vi "Zufalls(Musik-)auswahl.vi"() -> ()   [LabVIEW 2010]
uses:
  <vilib>/gmath/statdist.llb/Random Permutation.vi
  <vilib>/gmath/NI_Gmath.lvlib
panel:
  in  "start":i32 caption="Start"
  out "ausgelassene":i32
  out "wiederholungen":i32
  in  "seed":i32 caption="Startwert"
  in  "reset":bool caption="Zurücksetzen"
  in  "Playlist 2":i32(listbox) caption="Playlist"
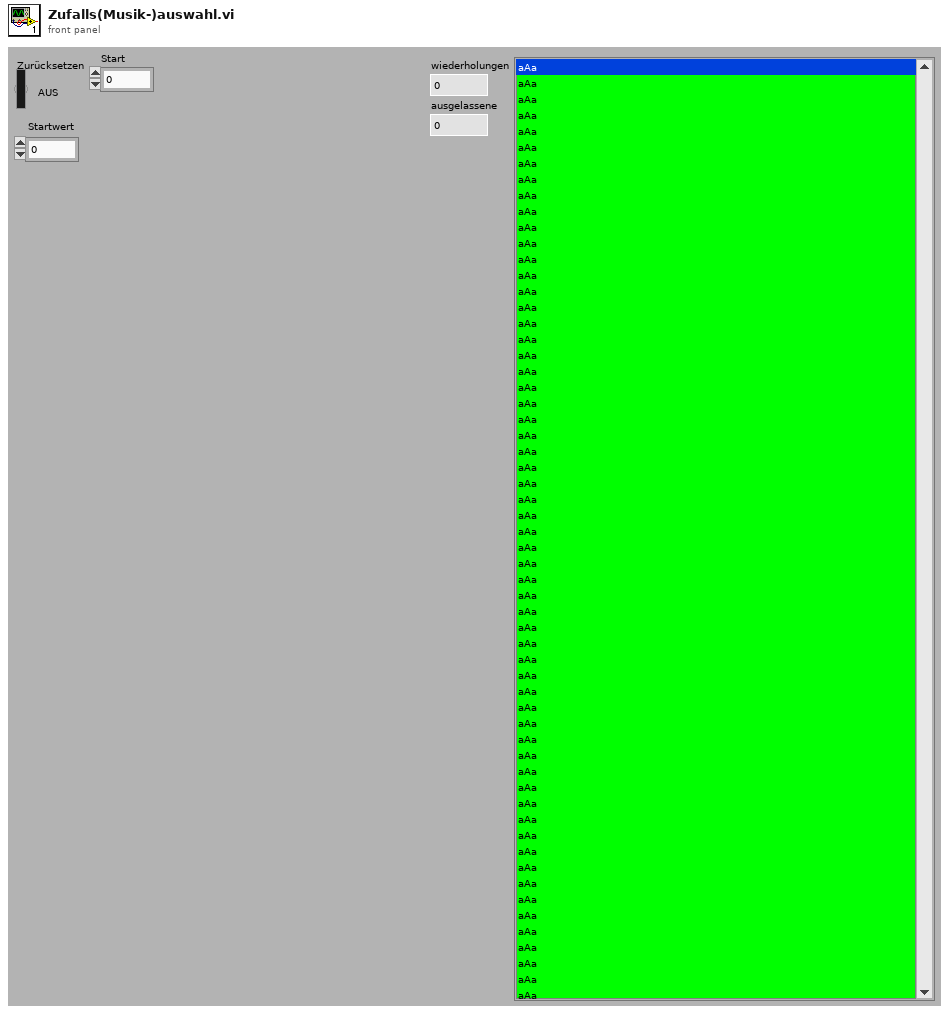
[diagram p1: front panel]
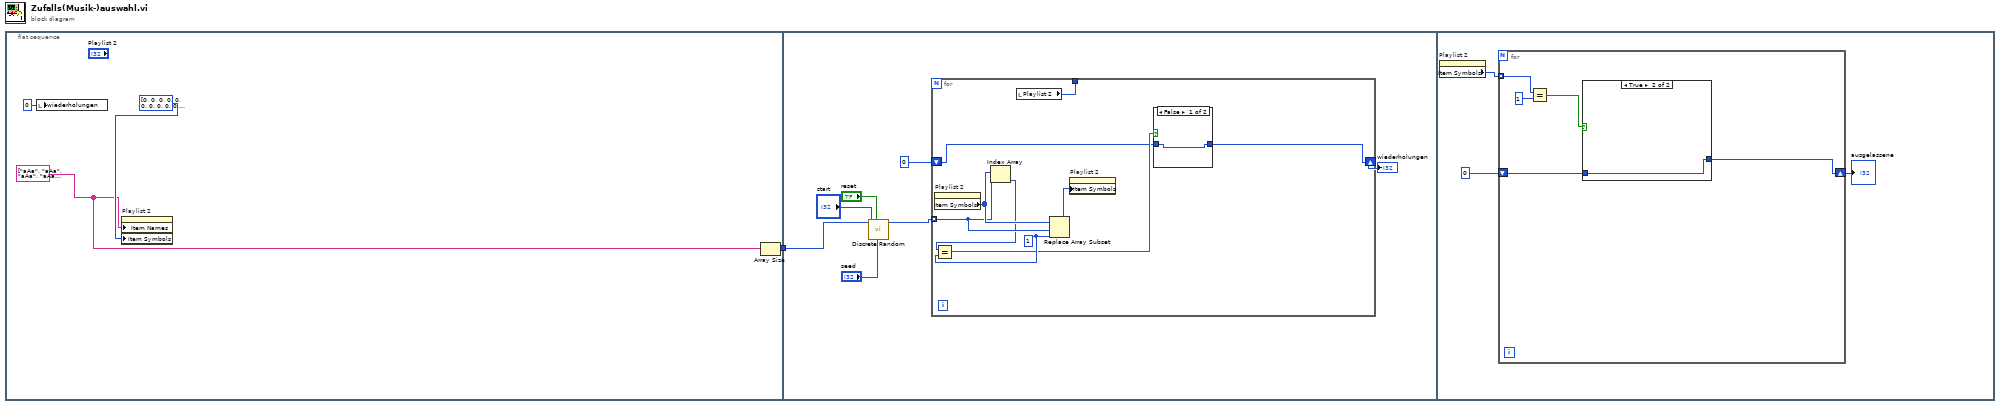
[diagram p0: block diagram]
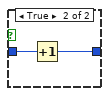
[diagram p2: hidden frame]
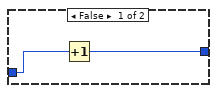
[diagram p3: hidden frame]
diagram:
  n1 = flat-sequence {
    tunnel: [w5] -> w1
    tunnel: w1 -> [w7]
    frame #0 {
      w2 = string[] ["aAa", "aAa", "aAa", "aAa", "aAa", "aAa", "aAa", "aAa", "aAa", "aAa", "aAa", "aAa", "aAa", "aAa", "aAa", "aAa", "aAa", "aAa", "aAa", "aAa", "aAa", "aAa", "aAa", "aAa", "aAa", "aAa", "aAa", "aAa", "aAa", "aAa", "aAa", "aAa", "aAa", "aAa", "aAa", "aAa", "aAa", "aAa", "aAa", "aAa", "aAa", "aAa", "aAa", "aAa", "aAa", "aAa", "aAa", "aAa", "aAa", "aAa", "aAa", "aAa", "aAa", "aAa", "aAa", "aAa", "aAa", "aAa", "aAa", "aAa", "aAa", "aAa", "aAa", "aAa", "aAa", "aAa", "aAa", "aAa", "aAa", "aAa", "aAa", "aAa", "aAa", "aAa", "aAa", "aAa", "aAa", "aAa", "aAa", "aAa", "aAa", "aAa", "aAa", "aAa", "aAa", "aAa", "aAa", "aAa", "aAa", "aAa", "aAa", "aAa", "aAa", "aAa", "aAa", "aAa", "aAa", "aAa", "aAa", "aAa", "aAa"] ("Item Names")
      n2 = local write "wiederholungen"(0 ("wiederholungen")) -> ()
      n3 = property on="Playlist 2" class="Listenfeld (strikt)"("Item Names"=w2, "Item Symbols"=i32[] [0, 0, 0, 0, 0, 0, 0, 0, 0, 0, 0, 0, 0, 0, 0, 0, 0, 0, 0, 0, 0, 0, 0, 0, 0, 0, 0, 0, 0, 0, 0, 0, 0, 0, 0, 0, 0, 0, 0, 0, 0, 0, 0, 0, 0, 0, 0, 0, 0, 0, 0, 0, 0, 0, 0, 0, 0, 0, 0, 0, 0, 0, 0, 0, 0, 0, 0, 0, 0, 0, 0, 0, 0, 0, 0, 0, 0, 0, 0, 0, 0, 0, 0, 0, 0, 0, 0, 0, 0, 0, 0, 0, 0, 0, 0, 0, 0, 0, 0, 0, 0]) -> ()  [unwired: 2 in, 2 out]
      n4 = Array Size(array=w2) -> (size(s)=w5:i32)
    }
    frame #1 {
      n5 = call-poly <vilib>:"Discrete Random.vi"("seed"="seed", "reset"="reset", "start"="start", "N"=w7) -> ("random permutation"=w12:i32[])  [unwired: 7 out]
      n6 = for {
        tunnel: w12 -> [w19] mode=indexing
        shift-right: [w14] -> w8
        shift-left: 0 -> [w15]
        tunnel: [w13] -> _
        w17 = 1 ("Neues Element/Teil-Array")
        n7 = property on="Playlist 2" class="Listenfeld (strikt)"() -> ("Item Symbols"=w20:i32[])  [unwired: 2 in, 2 out]
        n8 = Index Array(array=w20, index=w19) -> (element=w18:i32)
        n9 = Equal?(x=w18, y=w17) -> (x = y?=w16:bool)
        n10 = local read "Playlist 2"() -> (w13:i32)
        n11 = Replace Array Subset(array=w20, new element=w17, index=w19) -> (w21:i32[])
        n12 = property on="Playlist 2" class="Listenfeld (strikt)"("Item Symbols"=w21) -> ()  [unwired: 2 in, 2 out]
        n13 = case shown="False" w16 {
          tunnel: w15 -> [w22 w24]
          tunnel: [w22 w23] -> w14
          frame False {
          }
          frame True {
            n14 = Increment(x=w24) -> (x+1=w23:i32)
          }
        }
      }
      "wiederholungen" <- w8
    }
    frame #2 {
      n15 = property on="Playlist 2" class="Listenfeld (strikt)"() -> ("Item Symbols"=w27:i32[])  [unwired: 2 in, 2 out]
      n16 = for {
        tunnel: w27 -> [w32] mode=indexing
        shift-right: [w28] -> w25
        shift-left: 0 -> [w29]
        n17 = Equal?(x=w32, y=1) -> (x = y?=w30:bool)
        n18 = case shown="True" w30 {
          tunnel: w29 -> [w34 w35]
          tunnel: [w33 w35] -> w28
          frame False {
            n19 = Increment(x=w34) -> (x+1=w33:i32)
          }
          frame True {
          }
        }
      }
      "ausgelassene" <- w25
    }
  }
